vi "Save_Data.vi"(1 "Analysis Info cluster":T1[](array[typedef]) {"Sync Delay Time (s)" format="%.4f"; "Total Meas Time (s)" format="%_5g"; "Sd Error in Variance" format="%_3g"; "Skew_u" format="%_3g"; "% u'/U" format="%_3g"; "Sd Error in Mean" format="%_3g"; "Kurt_u" format="%_3g"; "u^4" format="%_3g"; "u^3" format="%_3g"; "U" format="%_3g"; "u^2" format="%_3g"}, 2 "Plot Data":cluster{"X array":dbl[], "Y array":dbl[]}, 3 "No of estimates output":i32=200, 4 "Index":u16, 5 "Weighting":dbl[](array[numeric]), 6 "Plot Type":T4=enum."Voltage trace") -> ()   [LabVIEW 2022 SP3]
uses:
  Controls/Graph_Type.ctl
  Controls/Analysis_info_cluster.ctl
  Controls/Inst_type.ctl
  Controls/Instrument_Array.ctl
  Controls/XY_Plot_Cluster.ctl
  File/File Update Cluster.ctl
  Globals/Meas_global.vi
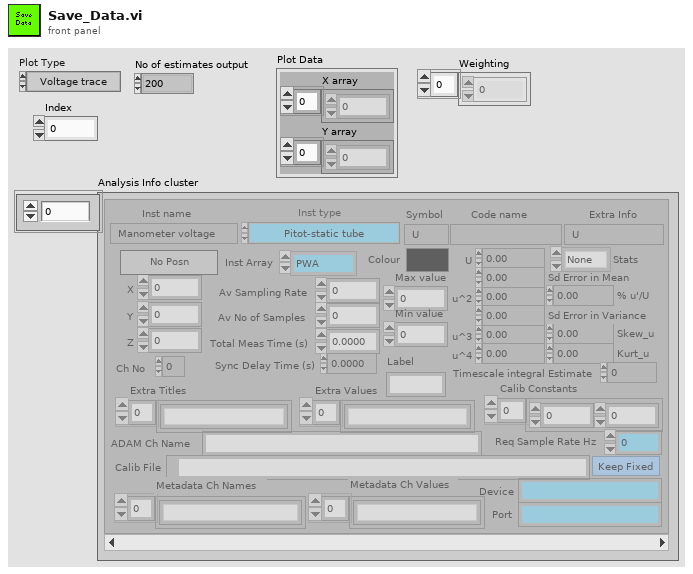
[diagram p1: front panel]
types:
  T1 = typedef "Analysis_info_cluster.ctl" = cluster{"Colour":u32, "Inst type":T2, "Inst name":string, "Symbol":string, "Code name":string, "Extra Info":string, "Inst Array":T3, "Extra Titles":string[], "Extra Values":string[], "U":dbl, "u^2":dbl, "u^3":dbl, "u^4":dbl, "Skew_u":dbl, "Kurt_u":dbl, "Sd Error in Mean":dbl, "% u'/U":dbl, "X":dbl, "Y":dbl, "Z":dbl, "Timescale integral Estimate":dbl, "Sd Error in Variance":dbl, "Calib File":path, "Calib Constants":dbl[], "Output Position":bool, "Stats":enum16{"None", "Basic", "Full"}, "Av Sampling Rate":dbl, "Av No of Samples":dbl, "Total Meas Time (s)":dbl, "ADAM Ch Name":string, "Max value":dbl, "Min value":dbl, "Req Sample Rate Hz":dbl, "Sync Delay Time (s)":dbl, "Ch No":i16, "Device":string, "Use Latest Calib":bool, "Port":string, "Metadata Ch Names":string[], "Metadata Ch Values":string[], "Label":string}
  T2 = typedef "Inst_type.ctl" = enum16{"Raw voltage", "Raw with zero offsetting", "Propeller anemometer", "Pressure Transducer", "Pitot-static tube", "Hot wire", "Cross wire 1", "Cross wire 2", "Generic Linear", "Generic Polynomial", "Generic BackPoly", "Fast FID", "Thermocouple", "Cold wire", "Pulsed Wire", "LDA Vel", "LDA Tran time", "LDA Arr time", "Microphone"}
  T3 = typedef "Instrument_Array.ctl" = enum16{"PWA", "LDA", "Analogue"}
  T4 = typedef "Graph_Type.ctl" = enum16{"Show no graph", "Voltage trace", "Velocity trace", "Vel histogram", "Spectrum", "f.E(f) v Log f", "Auto-Corr"}
  T5 = typedef "XY_Plot_Cluster.ctl" = cluster{"First Name":string, "Second Name":string, "X axis name":string, "Y axis name":string, "X array":dbl[], "Y array":dbl[], "Weighting":dbl[]}
  T6 = typedef "File Update Cluster.ctl" = cluster{"File Path":path, "Rows to Add":i32[], "Extra Ch Names":string[], "Extra Ch Values":string[], "Initial Header String":string, "Separation Character":enum16{"Tab", "Comma"}}
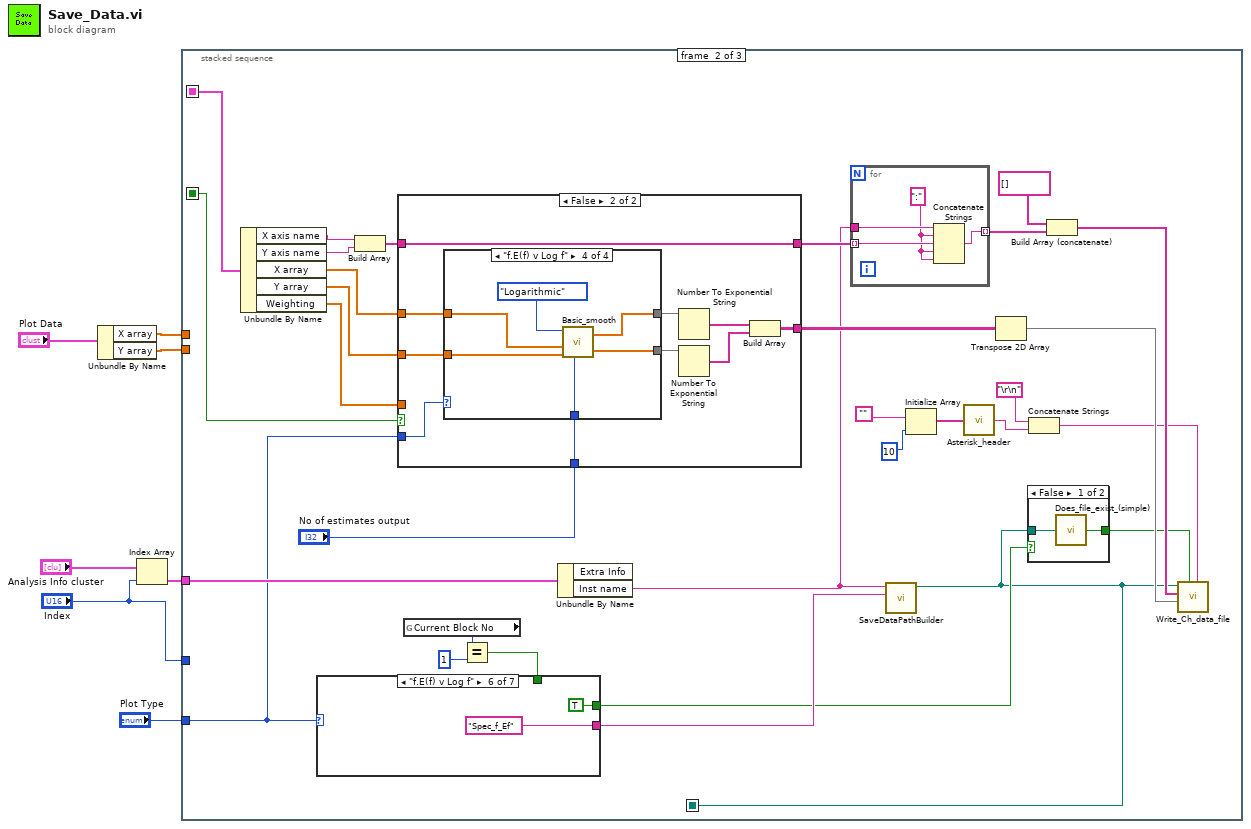
[diagram p0: block diagram]
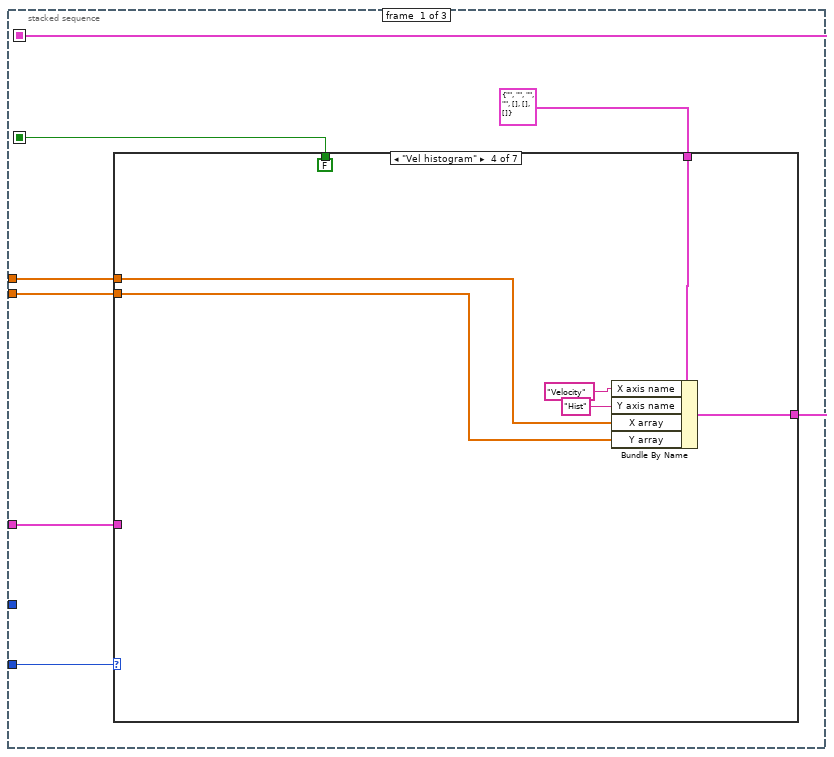
[diagram p2: hidden frame]
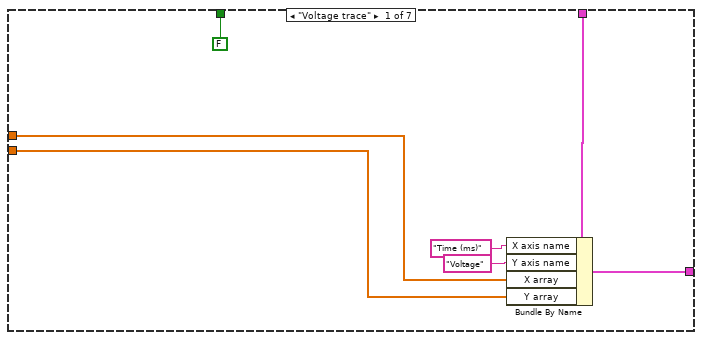
[diagram p3: hidden frame]
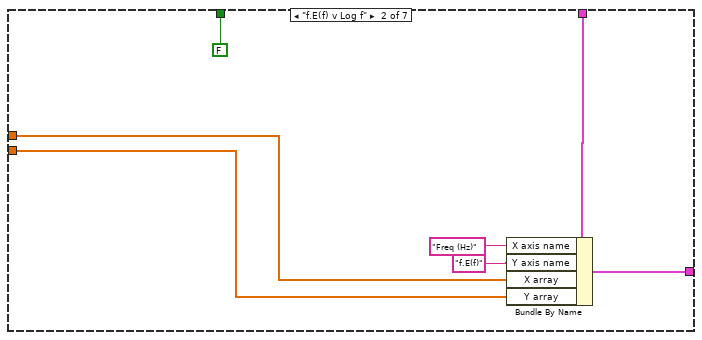
[diagram p4: hidden frame]
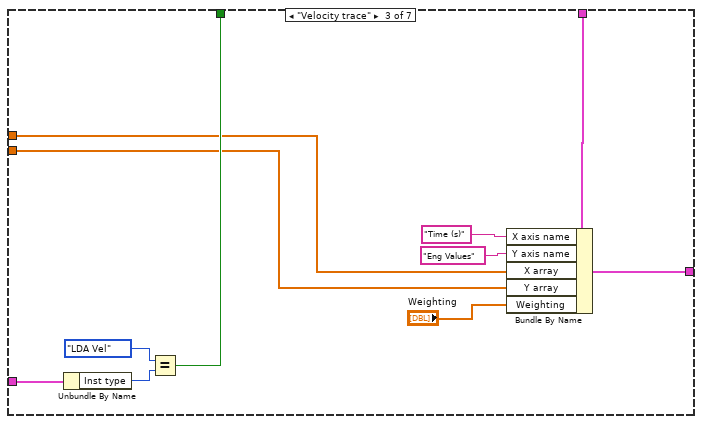
[diagram p5: hidden frame]
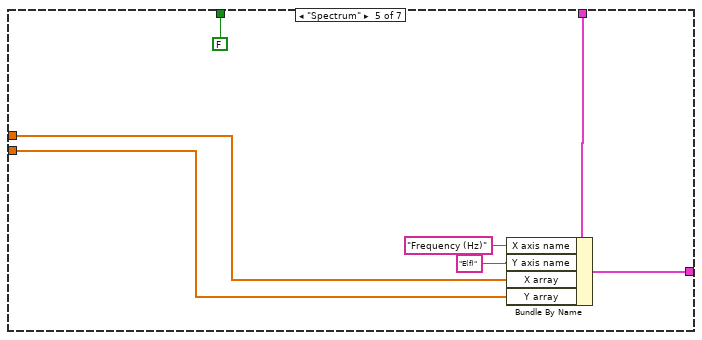
[diagram p6: hidden frame]
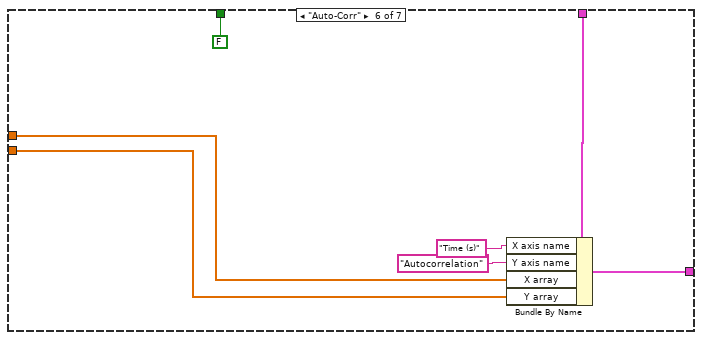
[diagram p7: hidden frame]
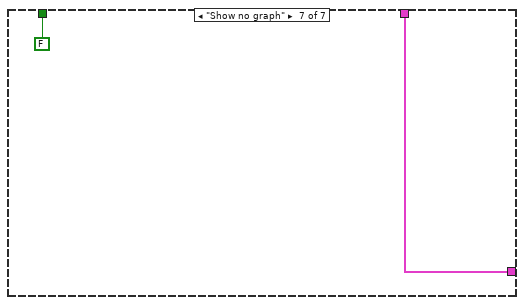
[diagram p8: hidden frame]
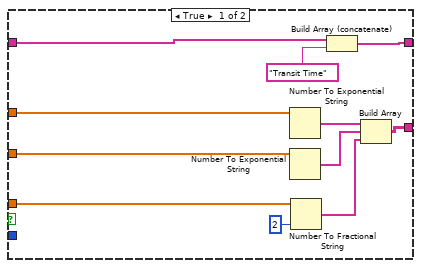
[diagram p9: hidden frame]
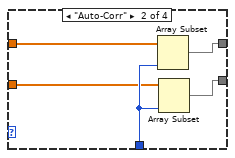
[diagram p11: hidden frame]
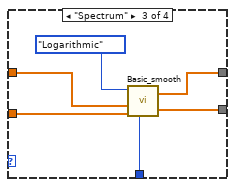
[diagram p12: hidden frame]
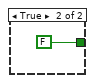
[diagram p13: hidden frame]
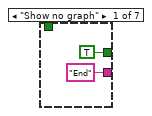
[diagram p14: hidden frame]
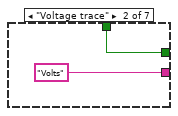
[diagram p15: hidden frame]
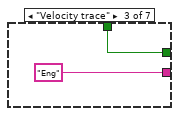
[diagram p16: hidden frame]
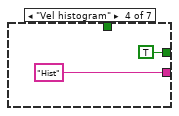
[diagram p17: hidden frame]
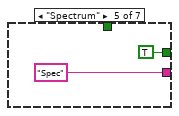
[diagram p18: hidden frame]
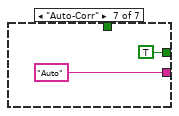
[diagram p19: hidden frame]
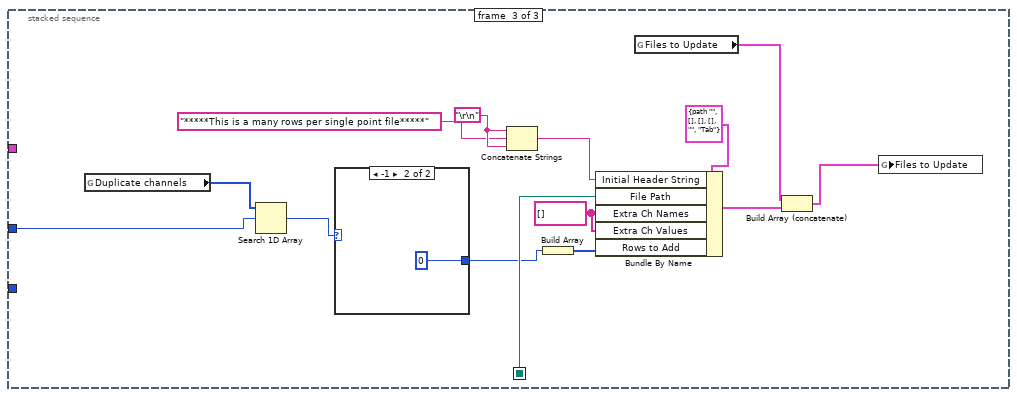
[diagram p20: hidden frame]
diagram:
  n1 = Unbundle By Name("Plot Data") -> ("X array"=w4:dbl[], "Y array"=w3:dbl[])
  n2 = Index Array(array="Analysis Info cluster", index="Index") -> (element=w6:T1)
  n3 = stacked-sequence {
    seq-local: [w12 _ _] -> [_ w82 _]
    seq-local: [w11 _ _] -> [_ w78 _]
    seq-local: [_ w69 _] -> [_ _ w163]
    tunnel: "Plot Type" -> [w14 w81 _]
    tunnel: w6 -> [w13 w88 _]
    tunnel: w4 -> [w9 _ _]
    tunnel: w3 -> [w8 _ _]
    tunnel: "Index" -> [_ _ w155]
    frame #0 {
      n4 = case shown="\"Vel histogram\"" w14 {
        tunnel: w13 -> [_ _ w39 _ _ _ _]
        tunnel: [w19 w26 w36 w42 w51 w54 w61] -> w12
        tunnel: [FALSE FALSE w33 FALSE FALSE FALSE FALSE] -> w11
        tunnel: T5 {"First Name"="", "Second Name"="", "X axis name"="", "Y axis name"="", "X array"=[], "Y array"=[], "Weighting"=[]} ("Spectra") -> [w17 w23 w32 w43 w52 w55 w61]
        tunnel: w9 -> [w16 w24 w30 w41 w50 w57 _]
        tunnel: w8 -> [w15 w22 w29 w40 w49 w56 _]
        frame "Voltage trace" {
          n5 = Bundle By Name(cluster=w17, "X axis name"="Time (ms)", "Y axis name"="Voltage", "X array"=w16, "Y array"=w15) -> (w19:T5)
        }
        frame "f.E(f) v Log f" {
          n6 = Bundle By Name(cluster=w23, "X axis name"="Freq (Hz)", "Y axis name"="f.E(f)", "X array"=w24, "Y array"=w22) -> (w26:T5)
        }
        frame "Velocity trace" {
          n7 = Unbundle By Name(w39) -> ("Inst type"=w35:T2)
          n8 = Equal?(x=Inst_type."LDA Vel" ("Inst type"), y=w35) -> (x = y?=w33:bool)
          n9 = Bundle By Name(cluster=w32, "X axis name"="Time (s)", "Y axis name"="Eng Values", "X array"=w30, "Y array"=w29, "Weighting"="Weighting") -> (w36:T5)
        }
        frame "Vel histogram" {
          n10 = Bundle By Name(cluster=w43, "X axis name"="Velocity", "Y axis name"="Hist", "X array"=w41, "Y array"=w40) -> (w42:T5)
        }
        frame "Spectrum" {
          n11 = Bundle By Name(cluster=w52, "X axis name"="Frequency (Hz)", "Y axis name"="E(f)", "X array"=w50, "Y array"=w49) -> (w51:T5)
        }
        frame "Auto-Corr" {
          n12 = Bundle By Name(cluster=w55, "X axis name"="Time (s)", "Y axis name"="Autocorrelation", "X array"=w57, "Y array"=w56) -> (w54:T5)
        }
        frame "Show no graph" {
        }
      }
    }
    frame #1 {
      n13 = Unbundle By Name(w82) -> ("X axis name"=w75:string, "Y axis name"=w74:string, "X array"=w80:dbl[], "Y array"=w79:dbl[], "Weighting"=w77:dbl[])
      n14 = Build Array(w75, w74) -> (w72:string[])
      n15 = case shown="False" w78 {
        tunnel: [w108 w118] -> w90
        tunnel: w81 -> [_ w116]
        tunnel: w80 -> [w106 w115]
        tunnel: w79 -> [w105 w114]
        tunnel: w77 -> [w103 _]
        tunnel: [w100 w110] -> w73
        tunnel: w72 -> [w101 w110]
        tunnel: "No of estimates output" -> [_ w109]
        frame True {
          n16 = Number To Exponential String(number=w106) -> (E-format string=w104:string[])  [unwired: 3 in]
          n17 = Number To Exponential String(number=w105) -> (E-format string=w107:string[])  [unwired: 3 in]
          n18 = Number To Fractional String(number=w103, precision (6)=i16 2) -> (F-format string=w102:string[])  [unwired: 2 in]
          n19 = Build Array (concatenate)(w101, "Transit Time") -> (w100:string[])
          n20 = Build Array(w104, w107, w102) -> (w108:string[][])
        }
        frame False {
          n21 = case shown="\"f.E(f) v Log f\"" w116 {
            tunnel: [w120 w123 w129 w135] -> w112
            tunnel: w115 -> [w120 w124 w131 w137]
            tunnel: w114 -> [w119 w122 w130 w136]
            tunnel: [w119 w121 w128 w134] -> w113
            tunnel: w109 -> [_ w125 w126 w132]
            frame "Voltage trace", Default {
            }
            frame "Auto-Corr" {
              n22 = Array Subset(array=w124, length=w125) -> (w123:dbl[])  [unwired: 1 in]
              n23 = Array Subset(array=w122, length=w125) -> (w121:dbl[])  [unwired: 1 in]
            }
            frame "Spectrum" {
              n24 = call "Basic_smooth.vi"("Smoothing"=enum16{"Linear", "Logarithmic"}."Logarithmic", "X array in"=w131, "Y array in"=w130, "No of estimates output"=w126) -> ("X array Out"=w129:dbl[], "Y array Out"=w128:dbl[])  [unwired: 1 out]
            }
            frame "f.E(f) v Log f" {
              n25 = call "Basic_smooth.vi"("Smoothing"=enum16{"Linear", "Logarithmic"}."Logarithmic", "X array in"=w137, "Y array in"=w136, "No of estimates output"=w132) -> ("X array Out"=w135:dbl[], "Y array Out"=w134:dbl[])  [unwired: 1 out]
            }
          }
          n26 = Number To Exponential String(number=w112) -> (E-format string=w111:string[])  [unwired: 3 in]
          n27 = Number To Exponential String(number=w113) -> (E-format string=w117:string[])  [unwired: 3 in]
          n28 = Build Array(w111, w117) -> (w118:string[][])
        }
      }
      n29 = global read "Meas_global.vi" "Current Block No"() -> (w86:i32)
      n30 = Equal?(x=w86, y=1) -> (x = y?=w83:bool)
      n31 = case shown="\"f.E(f) v Log f\"" w81 {
        tunnel: ["End" "Volts" "Eng" "Hist" "Spec" "Spec_f_Ef" "Auto"] -> w89
        tunnel: [TRUE w143 w145 TRUE TRUE TRUE TRUE] -> w84
        tunnel: w83 -> [_ w143 w145 _ _ _ _]
        frame "Show no graph" {
        }
        frame "Voltage trace" {
        }
        frame "Velocity trace" {
        }
        frame "Vel histogram" {
        }
        frame "Spectrum" {
        }
        frame "f.E(f) v Log f" {
        }
        frame "Auto-Corr" {
        }
      }
      n32 = Unbundle By Name(w88) -> ("Inst name"=w70:string)  [unwired: 1 out]
      n33 = for {
        tunnel: w70 -> [w97]
        tunnel: [w96] -> w76 mode=indexing
        tunnel: w73 -> [w95] mode=indexing
        w94 = ":" ("string")
        n34 = Concatenate Strings(w97, w94, w95, w94, w94) -> (w96:string)
      }
      n35 = call "SaveDataPathBuilder.vi"("DataTypeSuffix"=w89, "Inst name"=w70) -> ("Path name Out"=w69:path)  [unwired: 9 in]
      n36 = Initialize Array("", 10) -> (w68:string[])
      n37 = call "Asterisk_header.vi"("Channel names"=w68) -> ("Header string"=w64:string)
      n38 = Transpose 2D Array(2D array=w90) -> (transposed array=w91:string[][])
      n39 = case shown="False" w84 {
        tunnel: [w139 FALSE] -> w87
        tunnel: w69 -> [w138 _]
        frame False {
          n40 = call "Does_file_exist_(simple).vi"("Pathname"=w138) -> ("exists?"=w139:bool)
        }
        frame True {
        }
      }
      n41 = Concatenate Strings("\r\n", w64) -> (w63:string)
      n42 = Build Array (concatenate)(string[] [], w76) -> (w92:string[])
      n43 = call "Write_Ch_data_file.vi"("Header string"=w63, "exists?"=w87, "Channel Values"=w91, "Channel names"=w92, "Filename"=w69) -> ()  [unwired: 2 in, 5 out]
    }
    frame #2 {
      w164 = string[] [] ("Extra Ch Names")
      w167 = "\r\n"
      n44 = global read "Meas_global.vi" "Duplicate channels"() -> (w159:i32[])
      n45 = Search 1D Array(1D array=w159, element=w155) -> (index of element=w158:i32)  [unwired: 1 in]
      n46 = case shown="-1" w158 {
        selector: w158 -> [w169 _]
        tunnel: [w169 0 ("Rows to Add")] -> w156
        frame 0, Default {
        }
        frame -1 {
        }
      }
      n47 = Concatenate Strings(w167, "*****This is a many rows per single point file*****", w167) -> (w168:string)
      n48 = Build Array(w156) -> (w157:i32[])
      n49 = Bundle By Name(cluster=T6 {"File Path"=path "", "Rows to Add"=[], "Extra Ch Names"=[], "Extra Ch Values"=[], "Initial Header String"="", "Separation Character"=enum."Tab"} ("File to Update"), "Initial Header String"=w168, "File Path"=w163, "Extra Ch Names"=w164, "Extra Ch Values"=w164, "Rows to Add"=w157) -> (w162:T6)
      n50 = global read "Meas_global.vi" "Files to Update"() -> (w161:T6[])
      n51 = Build Array (concatenate)(w161, w162) -> (w160:T6[])
      n52 = global write "Meas_global.vi" "Files to Update"(w160) -> ()
    }
  }
